vi "programComm.vi"(1 "error in (no error)":errorcluster, 2 "CommSelect":T1(ring)) -> (0 "error out":errorcluster)   [LabVIEW 2014]
uses:
  GlobComm.vi
panel:
  out "commData4Button":u32[](array[numeric])=[4278190080, 3149642683, 3435973836, 3722304989, 4008636142, 4294967295, 10, 10, 10, 10, 10, 10, 10, 10, 10, 10, 10, 10, 10, 10, 10, 10, 10, 10, 10, 10, 10, 10, 10, 10, 10, 10] format="%b"
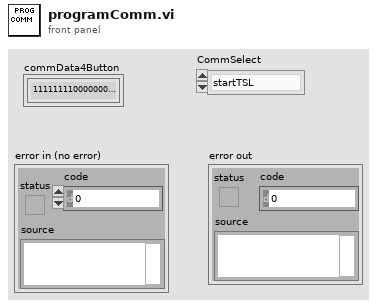
[diagram p1: front panel]
types:
  T1 = enum16{"startTSL", "writeCABAC", "readCABAC", "resetCABAC", "emissionTest", "regRead", "executeASPIC", "resetASPIC", "resetFifo18ASPIC", "resetFifo16ASPIC", "LabviewDamicStart"}
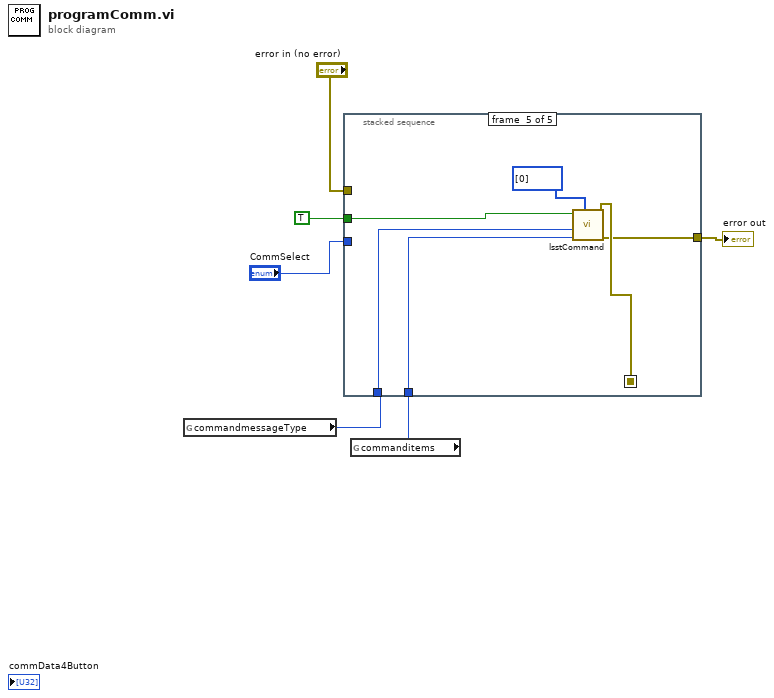
[diagram p0: block diagram]
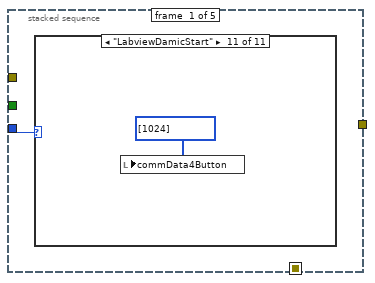
[diagram p2: hidden frame]
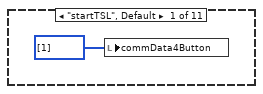
[diagram p3: hidden frame]
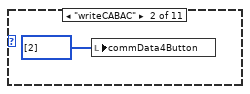
[diagram p4: hidden frame]
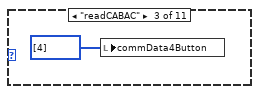
[diagram p5: hidden frame]
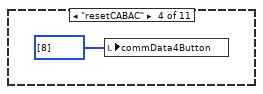
[diagram p6: hidden frame]
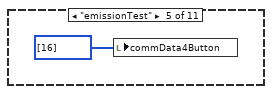
[diagram p7: hidden frame]
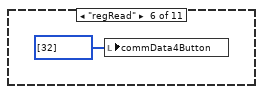
[diagram p8: hidden frame]
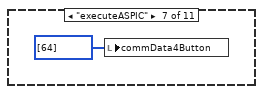
[diagram p9: hidden frame]
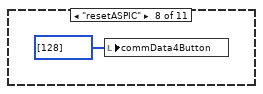
[diagram p10: hidden frame]
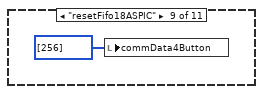
[diagram p11: hidden frame]
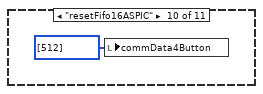
[diagram p12: hidden frame]
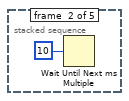
[diagram p13: hidden frame]
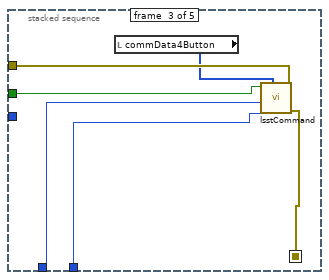
[diagram p14: hidden frame]
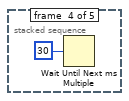
[diagram p15: hidden frame]
diagram:
  n1 = global read "GlobComm.vi" "commandmessageType"() -> (w5:u32)
  n2 = global read "GlobComm.vi" "commanditems"() -> (w4:u8)
  n3 = stacked-sequence {
    seq-local: [_ _ w20 _ _] -> [_ _ _ _ w28]
    tunnel: w5 -> [_ _ w25 _ w31]
    tunnel: "error in (no error)" -> [_ _ w24 _ _]
    tunnel: w4 -> [_ _ w23 _ w30]
    tunnel: TRUE ("execute") -> [_ _ w22 _ w29]
    tunnel: "CommSelect" -> [w7 _ _ _ _]
    tunnel: [_ _ _ _ w27] -> w1
    frame #0 {
      n4 = case shown="\"LabviewDamicStart\"" w7 {
        frame "startTSL", Default {
          n5 = local write "commData4Button"(u32[] [1] ("data")) -> ()
        }
        frame "writeCABAC" {
          n6 = local write "commData4Button"(u32[] [2] ("data")) -> ()
        }
        frame "readCABAC" {
          n7 = local write "commData4Button"(u32[] [4] ("data")) -> ()
        }
        frame "resetCABAC" {
          n8 = local write "commData4Button"(u32[] [8] ("data")) -> ()
        }
        frame "emissionTest" {
          n9 = local write "commData4Button"(u32[] [16] ("data")) -> ()
        }
        frame "regRead" {
          n10 = local write "commData4Button"(u32[] [32] ("data")) -> ()
        }
        frame "executeASPIC" {
          n11 = local write "commData4Button"(u32[] [64] ("data")) -> ()
        }
        frame "resetASPIC" {
          n12 = local write "commData4Button"(u32[] [128] ("data")) -> ()
        }
        frame "resetFifo18ASPIC" {
          n13 = local write "commData4Button"(u32[] [256] ("data")) -> ()
        }
        frame "resetFifo16ASPIC" {
          n14 = local write "commData4Button"(u32[] [512] ("data")) -> ()
        }
        frame "LabviewDamicStart" {
          n15 = local write "commData4Button"(u32[] [1024] ("data")) -> ()
        }
      }
    }
    frame #1 {
      n16 = Wait Until Next ms Multiple(millisecond multiple=u32 10 ("millisecond timer value")) -> ()  [unwired: 1 out]
    }
    frame #2 {
      n17 = local read "commData4Button"() -> (w21:u32[])
      n18 = call "lsstCommand.vi"("error in (no error)"=w24, "data"=w21, "nbitems"=w23, "messagetype"=w25, "execute"=w22) -> ("error out"=w20:errorcluster)  [unwired: 2 in, 4 out]
    }
    frame #3 {
      n19 = Wait Until Next ms Multiple(millisecond multiple=u32 30 ("millisecond timer value")) -> ()  [unwired: 1 out]
    }
    frame #4 {
      n20 = call "lsstCommand.vi"("error in (no error)"=w28, "data"=u32[] [0], "nbitems"=w30, "messagetype"=w31, "execute"=w29) -> ("error out"=w27:errorcluster)  [unwired: 2 in, 4 out]
    }
  }
  "error out" <- w1
